vi "init.vi"() -> (0 "success":bool)   [LabVIEW 2012]
uses:
  <userlib>/atmcd32d.llb/Error Code Enum typedef.ctl
  <userlib>/atmcd32d.llb/AcquisitionMode_mode typedef.ctl
  <userlib>/atmcd32d.llb/Spool_method typedef.ctl
  <userlib>/atmcd32d.llb/Shutter_mode typedef.ctl
  <userlib>/atmcd32d.llb/Shutter_type typedef.ctl
  <userlib>/atmcd32d.llb/TriggerMode_mode typedef.ctl
panel:
  out "Return from Initialize":u32
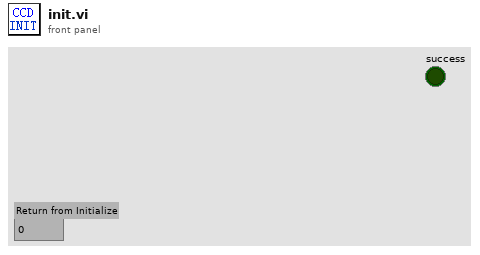
[diagram p1: front panel]
types:
  T1 = typedef "Error Code Enum typedef.ctl" = enum32{"N/A (0)", "DRV_ERROR_CODES", "DRV_SUCCESS", "DRV_VXDNOTINSTALLED", "DRV_ERROR_SCAN", "DRV_ERROR_CHECK_SUM", "DRV_ERROR_FILELOAD", "DRV_UNKNOWN_FUNC", "DRV_ERROR_VXD_INIT", "DRV_ERROR_ADDRESS", "DRV_ERROR_PAGELOCK", "DRV_ERROR_PAGEUNLOCK", "DRV_ERROR_BOARDTEST", "DRV_ERROR_ACK", "DRV_ERROR_UP_FIFO", "DRV_ERROR_PATTERN", "N/A (16)", "DRV_ACQUISITION_ERRORS", "DRV_ACQ_BUFFER", "DRV_ACQ_DOWNFIFO_FULL", "DRV_PROC_UNKONWN_INSTRUCTION", "DRV_ILLEGAL_OP_CODE", "DRV_KINETIC_TIME_NOT_MET", "DRV_ACCUM_TIME_NOT_MET", "DRV_NO_NEW_DATA", "N/A (25)", "DRV_SPOOLERROR", "N/A (27)", "N/A (28)", "N/A (29)", "N/A (30)", "N/A (31)", "N/A (32)", "DRV_TEMPERATURE_CODES", "DRV_TEMPERATURE_OFF", "DRV_TEMPERATURE_NOT_STABILIZED", "DRV_TEMPERATURE_STABILIZED", "DRV_TEMPERATURE_NOT_REACHED", "DRV_TEMPERATURE_OUT_RANGE", "DRV_TEMPERATURE_NOT_SUPPORTED", "DRV_TEMPERATURE_DRIFT", "N/A (41)", "N/A (42)", "N/A (43)", "N/A (44)", "N/A (45)", "N/A (46)", "N/A (47)", "N/A (48)", "DRV_GENERAL_ERRORS", "DRV_INVALID_AUX", "DRV_COF_NOTLOADED", "DRV_FPGAPROG", "DRV_FLEXERROR", "DRV_GPIBERROR", "N/A (55)", "N/A (56)", "N/A (57)", "N/A (58)", "N/A (59)", "N/A (60)", "N/A (61)", "N/A (62)", "N/A (63)", "DRV_DATATYPE", "DRV_DRIVER_ERRORS", "DRV_P1INVALID", "DRV_P2INVALID", "DRV_P3INVALID", "DRV_P4INVALID", "DRV_INIERROR", "DRV_COFERROR", "DRV_ACQUIRING", "DRV_IDLE", "DRV_TEMPCYCLE", "DRV_NOT_INITIALIZED", "DRV_P5INVALID", "DRV_P6INVALID", "DRV_INVALID_MODE", "DRV_INVALID_FILTER", "DRV_I2CERRORS", "DRV_I2CDEVNOTFOUND", "DRV_I2CTIMEOUT", "DRV_P7INVALID", "N/A (84)", "N/A (85)", "N/A (86)", "N/A (87)", "N/A (88)", "N/A (89)", "DRV_IOCERROR", "DRV_VRMVERSIONERROR"}
  T2 = typedef "AcquisitionMode_mode typedef.ctl" = enum16{"Reserved (0)", "Single Scan", "Accumulate", "Kinetics", "Fast Kinetics", "Run Till Abort", "Reserved (6)", "Reserved (7)", "Reserved (8)", "Time Delayed Integration"}
  T3 = typedef "Spool_method typedef.ctl" = enum16{"32-bit", "Depends", "16-bit", "Multiple Directory", "Spool to RAM disk", "16-bit FITS", "SIF", "16-buit TIFF", "Multiple Directory Compressed"}
  T4 = typedef "Shutter_type typedef.ctl" = enum16{"TTL Low", "TTL High"}
  T5 = typedef "Shutter_mode typedef.ctl" = enum16{"Auto", "Open", "Close"}
  T6 = typedef "TriggerMode_mode typedef.ctl" = enum16{"Internal", "External", "N/A (2)", "N/A (3)", "N/A (4)", "N/A (5)", "External Start", "External Exposure (Bulb)", "N/A (8)", "External FVB EM", "Software", "N/A (11)", "External Charge Shifting"}
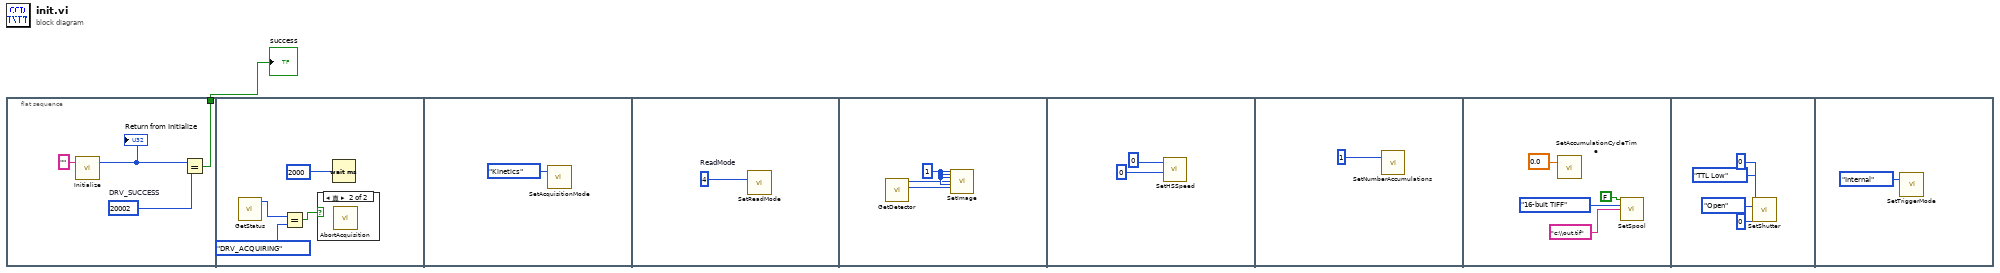
[diagram p0: block diagram]
diagram:
  n1 = flat-sequence {
    tunnel: [w2] -> w1
    frame #0 {
      w3 = 20002  # DRV_SUCCESS
      n2 = call <userlib>:"Initialize.vi"("directory (\"\")"="" ("directory (\"\")")) -> ("DLL error code"=w4:u32)  [unwired: 1 in, 1 out]
      "Return from Initialize" <- w4
      n3 = Equal?(x=w4, y=w3) -> (x = y?=w2:bool)
    }
    frame #1 {
      n4 = call <userlib>:"GetStatus.vi"() -> ("status"=w8:T1)  [unwired: 3 in, 2 out]
      n5 = Equal?(x=w8, y=Error_Code_Enum_typedef."DRV_ACQUIRING") -> (x = y?=w6:bool)
      n6 = case shown="真" w6 {
        frame False {
        }
        frame True {
          n7 = call <userlib>:"AbortAcquisition.vi"() -> ()  [unwired: 2 in, 2 out]
        }
      }
      n8 = Wait (ms)(milliseconds to wait=u32 2000) -> ()  [unwired: 1 out]
    }
    frame #2 {
      n9 = call <userlib>:"SetAcquisitionMode.vi"("mode"=AcquisitionMode_mode_typedef."Kinetics") -> ()  [unwired: 1 in, 2 out]
    }
    frame #3 {
      w11 = u16 4  # ReadMode
      n10 = call <userlib>:"SetReadMode.vi"("mode"=w11) -> ()  [unwired: 1 in, 2 out]
    }
    frame #4 {
      w14 = 1
      n11 = call <userlib>:"GetDetector.vi"() -> ("ypixels"=w12:i32, "xpixels"=w13:i32)  [unwired: 4 in, 2 out]
      n12 = call <userlib>:"SetImage.vi"("hbin"=w14, "vbin"=w14, "hstart"=w14, "hend"=w13, "vstart"=w14, "vend"=w12) -> ()  [unwired: 20 in, 2 out]
    }
    frame #5 {
      n13 = call <userlib>:"SetHSSpeed.vi"("index"=0, "type"=0) -> ()  [unwired: 2 in, 2 out]
    }
    frame #6 {
      n14 = call <userlib>:"SetNumberAccumulations.vi"("number"=1) -> ()  [unwired: 1 in, 2 out]
    }
    frame #7 {
      n15 = call <userlib>:"SetAccumulationCycleTime.vi"("time"=sgl 0.0) -> ()  [unwired: 1 in, 2 out]
      n16 = call <userlib>:"SetSpool.vi"("active"=FALSE, "method"=Spool_method_typedef."16-buit TIFF", "name"="c:\\out.tif") -> ()  [unwired: 11 in, 2 out]
    }
    frame #8 {
      n17 = call <userlib>:"SetShutter.vi"("type"=Shutter_type_typedef."TTL Low", "mode"=Shutter_mode_typedef."Open", "closingtime"=0, "openingtime"=0) -> ()  [unwired: 10 in, 2 out]
    }
    frame #9 {
      n18 = call <userlib>:"SetTriggerMode.vi"("mode"=TriggerMode_mode_typedef."Internal") -> ()  [unwired: 1 in, 2 out]
    }
  }
  "success" <- w1
